vi "MC Data queue generator.vi"(8 "error in (no error)":errorcluster) -> (0 "error out":errorcluster)   [LabVIEW 2020]
uses:
  templates/Queue Access FGV/Controls/FGV State Command.ctl
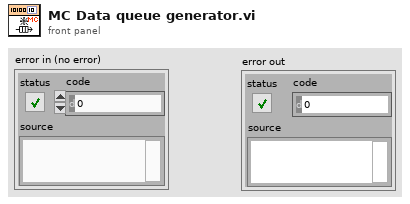
[diagram p1: front panel]
types:
  T1 = typedef "FGV State Command.ctl" = enum16{"Get", "Initialize", "Release"}
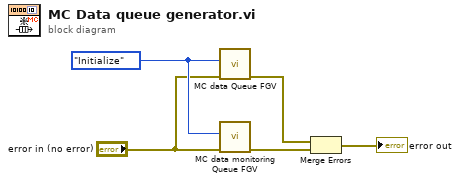
[diagram p0: block diagram]
diagram:
  w4 = FGV_State_Command."Initialize" ("FGV State Command")
  n1 = call "MC data Queue FGV.vi"("FGV State Command"=w4, "error in (no error)"="error in (no error)") -> ("error out"=w2:errorcluster)  [unwired: 7 in, 1 out]
  n2 = call "MC data monitoring Queue FGV.vi"("FGV State Command"=w4, "error in (no error)"="error in (no error)") -> ("error out"=w1:errorcluster)  [unwired: 7 in, 1 out]
  n3 = Merge Errors(w2, w1) -> (→"error out":errorcluster)
